vi "Stream Data.vi"(8 "Error In":errorcluster, 10 "Data Type":string, 11 "Communication In":refnum<class "Communication.lvclass">) -> (0 "Error Out":errorcluster, 3 "Communication Out":refnum<class "Communication.lvclass">)   [LabVIEW 2022 SP3, in "Communication.lvclass"]
doc: "This VI is an overriding method of parent data class which gets the data for streaming data."
uses:
  Communication.lvclass
  Data/Data.lvclass
  Controls/User Event Operation.ctl
  Downloads/Sample PC Template/Sample PC Template/Typedefs/Data.ctl
  Downloads/Sample PC Template/Sample PC Template/Sample PC Template.lvlib
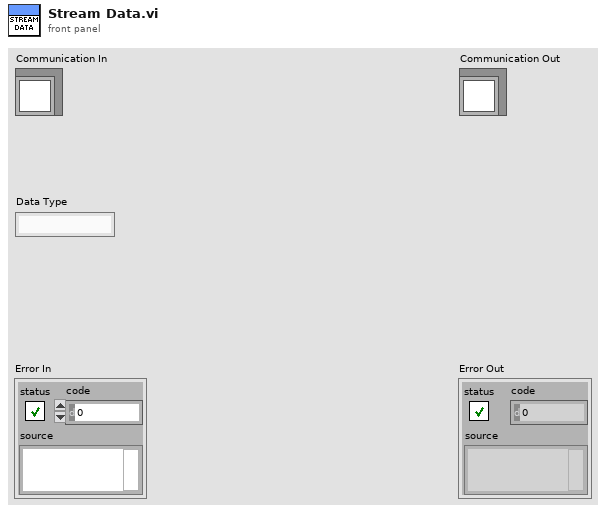
[diagram p1: front panel]
types:
  T1 = typedef "Sample PC Template.lvlib/Data.ctl" = cluster{"State":string, "Data":variant}
  T2 = typedef "User Event Operation.ctl" = enum16{"Obtain", "Generate", "Release"}
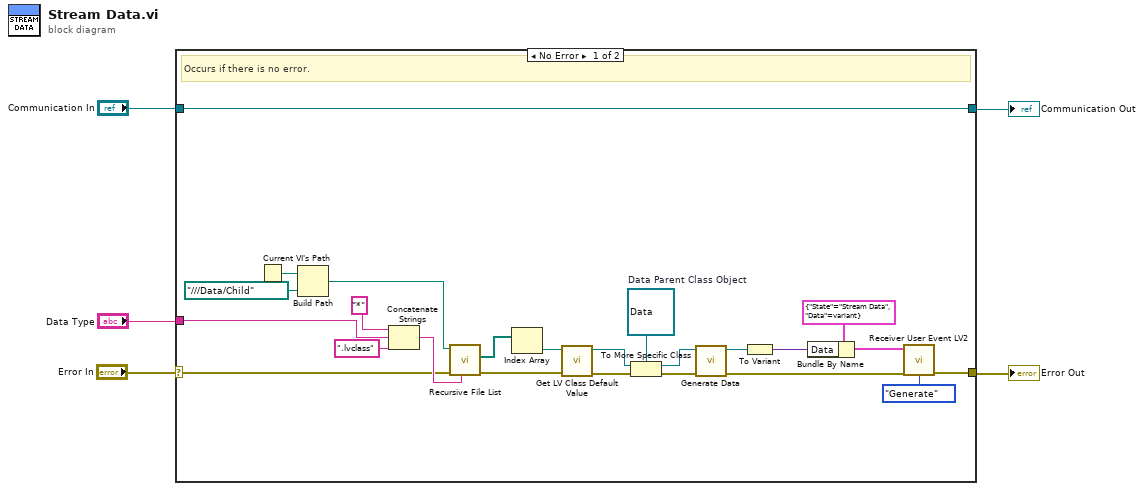
[diagram p0: block diagram]
diagram:
  n1 = case shown="No Error" "Error In" {
    selector: "Error In" -> [w10 w31]
    tunnel: [w9 w31] -> w4
    tunnel: [w29 w30] -> w2
    tunnel: "Communication In" -> [w29 w30]
    tunnel: "Data Type" -> [w8 _]
    frame No Error {
      w23 = refnum<class "Data.lvclass"> refnum  # Data Parent Class Object
      # "Occurs if there is no error."
      n2 = Current VI's Path() -> (path=w28:path)
      n3 = Build Path(base path=w28, name or relative path=path "../../../Data/Child") -> (appended path=w15:path)
      n4 = Concatenate Strings("*" ("string"), w8, ".lvclass" ("string")) -> (w12:string)
      n5 = call <vilib>:"Recursive File List.vi"("pattern"=w12, "error in (no error)"=w10, "Folder Path"=w15) -> ("error out"=w27:errorcluster, "All Files in Dir"=w26:path[])  [unwired: 4 in, 3 out]
      n6 = Index Array(array=w26) -> (element=w11:path)  [unwired: 1 in]
      n7 = call <vilib>:"Get LV Class Default Value.vi"("error in (no error)"=w27, "class path"=w11) -> ("error out"=w24:errorcluster, "object"=w22:refnum<class>)  [unwired: 8 in]
      n8 = To More Specific Class(target class=w23, reference=w22, error in=w24) -> (specific class reference=w20:refnum<class "Data.lvclass">, error out=w21:errorcluster)
      n9 = call-dynamic "Generate Data.vi"("error in (no error)"=w21, "Data in"=w20) -> ("error out"=w19:errorcluster, "Data out"=w7:refnum<class "Data.lvclass">)  [unwired: 8 in]
      n10 = To Variant(anything=w7) -> (Variant=w6:variant)
      n11 = Bundle By Name(cluster=T1 {"State"="Stream Data", "Data"=variant} ("Data"), "Data"=w6) -> (w16:T1)
      n12 = call "Receiver User Event LV2.vi"("Data"=w16, "Error In"=w19, "Operation"=User_Event_Operation."Generate") -> ("Error Out"=w9:errorcluster)  [unwired: 11 in, 1 out]
    }
    frame Error {
      # "Occurs if there is any error."
    }
  }
  "Error Out" <- w4
  "Communication Out" <- w2
